vi "Wavefront Correction (SubVI).vi"(1 "Source Image Array":u8[](array[numeric]), 2 "Correction Path":path) -> (0 "Corrected Image Array":u8[](array[numeric]))   [LabVIEW 2010]
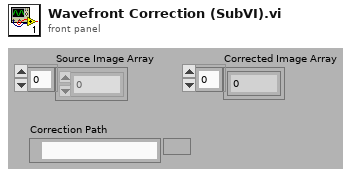
[diagram p1: front panel]
types:
  T1 = typedef "imagedata.ctl" = cluster{"image type":i32, "image depth":i32, "image":u8[], "mask":u8[], "colors":u32[], "Rectangle":cluster{"left":i16, "top":i16, "right":i16, "bottom":i16}}
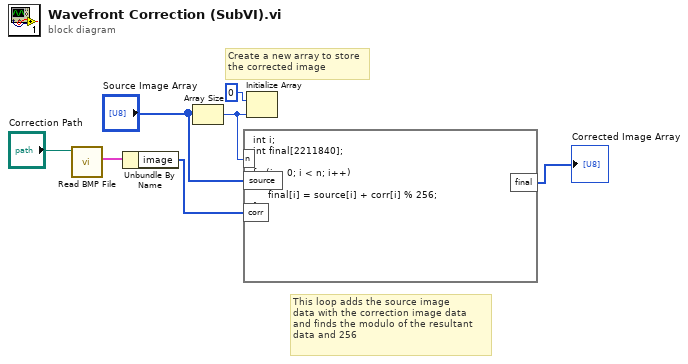
[diagram p0: block diagram]
diagram:
  # "This loop adds the source image\ndata with the correction image data\nand finds the modulo of the resultant\ndata and 256"
  # "Create a new array to store\nthe corrected image"
  n1 = call <vilib>:"Read BMP File.vi"("path to BMP file"="Correction Path") -> ("image data"=w6:T1)  [unwired: 8 in, 2 out]
  n2 = Unbundle By Name(w6) -> ("image"=w2:u8[])
  n3 = Array Size(array="Source Image Array") -> (size(s)=w4:i32)
  n4 = formula code="int i;\nint final[2211840];\n\nfor(i = 0; i < n; i++)\n{\n     final[i] = source[i] + corr[i] % 256;\n}"("n"=w4, "source"="Source Image Array", "corr"=w2) -> ("final"=→"Corrected Image Array":i32[])
  n5 = Initialize Array(u8 0, w4) -> ()  [unwired: 1 out]
